vi "buildTerminalName.vi"(8 "error in (no error)":errorcluster, 9 "Local Terminal Name":string="/Engine0/SourceCompleteEvent", 10 "Channel Name":string="0", 11 "session handle":refnum<k15>="4139_1") -> (0 "error IO":errorcluster, 2 "Fully Qualified Terminal Name":string="/4139_1/Engine//Engine0/SourceCompleteEvent", 3 "session handle 2":refnum<k15>="4139_1")   [LabVIEW 2014]
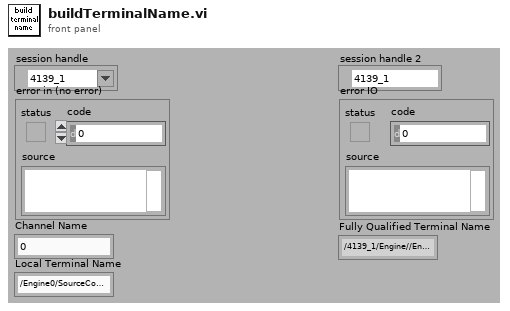
[diagram p1: front panel]
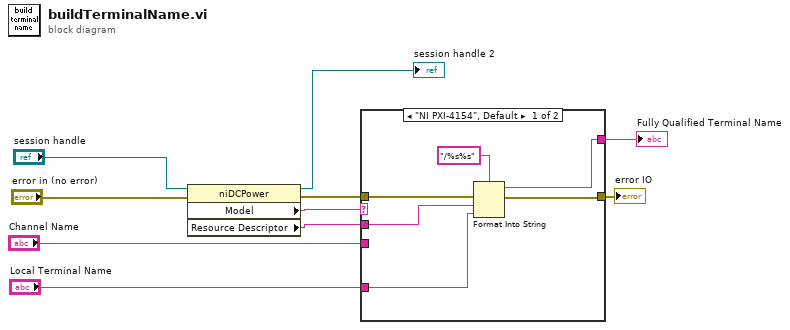
[diagram p0: block diagram]
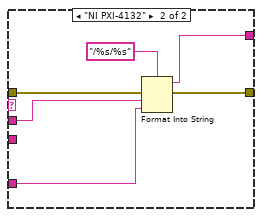
[diagram p2: hidden frame]
diagram:
  n1 = property class="niDCPower"(reference="session handle", error in="error in (no error)") -> (reference out=→"session handle 2":refnum<k15>, error out=w6:errorcluster, "Model"=w10:string, "Resource Descriptor"=w3:string)
  n2 = case shown="\"NI PXI-4154\", Default" w10 {
    tunnel: w6 -> [w16 w22]
    tunnel: [w15 w21] -> w5
    tunnel: [w14 w20] -> w4
    tunnel: w3 -> [w12 w18]
    tunnel: "Channel Name" -> [_ _]
    tunnel: "Local Terminal Name" -> [w11 w17]
    frame "NI PXI-4154", Default {
      n3 = Format Into String(format string="/%s%s", error in=w16, w12, w11) -> (resulting string=w14:string, error out=w15:errorcluster)  [unwired: 1 in]
    }
    frame "NI PXI-4132" {
      n4 = Format Into String(format string="/%s/%s", error in=w22, w18, w17) -> (resulting string=w20:string, error out=w21:errorcluster)  [unwired: 1 in]
    }
  }
  "error IO" <- w5
  "Fully Qualified Terminal Name" <- w4
